vi "Build Toolkit HTML Documentation.vi"(8 "Error In":errorcluster) -> (0 "Error Out":errorcluster)   [LabVIEW 2018, in "Scripts.lvlib"]
uses:
  Scripts.lvlib
  <vilib>/Field R&D Services/Labricator/Toolkit/Labricator.lvlib
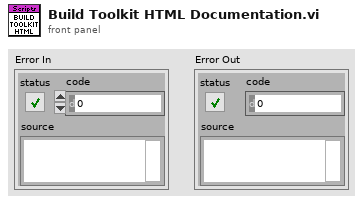
[diagram p1: front panel]
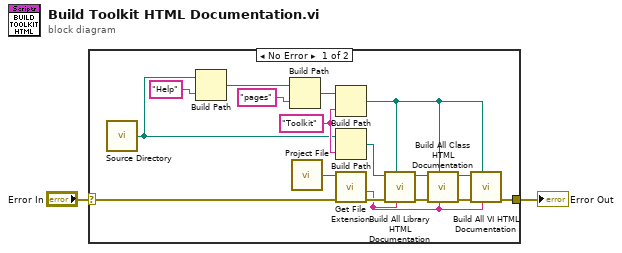
[diagram p0: block diagram]
diagram:
  n1 = case shown="No Error" "Error In" {
    selector: "Error In" -> [w14 w20]
    tunnel: [w17 w20] -> w1
    frame No Error {
      w7 = "Toolkit" ("name or relative path")
      n2 = call <vilib>:"Source Directory.vi"() -> ("Source Directory"=w5:path)
      n3 = Build Path(base path=w5, name or relative path="Help") -> (appended path=w10:path)
      n4 = Build Path(base path=w10, name or relative path="pages") -> (appended path=w8:path)
      n5 = call <vilib>:"Project File.vi"() -> ("Project File"=w15:path)
      n6 = Build Path(base path=w8, name or relative path=w7) -> (appended path=w6:path)
      n7 = Build Path(base path=w5, name or relative path=w7) -> (appended path=w16:path)
      n8 = call <vilib>:"Get File Extension.vi"("error in (no error)"=w14, "file"=w15) -> ("error out"=w13:errorcluster, "filename without extension"=w12:string)  [unwired: 5 in, 3 out]
      n9 = call "Build All Library HTML Documentation.vi"("Requirement"=w12, "Destination"=w6, "Error In"=w13, "Source In"=w16) -> ("Error Out"=w18:errorcluster, "Source Out"=w19:path)  [unwired: 6 in]
      n10 = call "Build All Class HTML Documentation.vi"("Requirement"=w12, "Destination"=w6, "Error In"=w18, "Source In"=w19) -> ("Error Out"=w3:errorcluster, "Source Out"=w4:path)  [unwired: 6 in]
      n11 = call "Build All VI HTML Documentation.vi"("Requirement"=w12, "Destination"=w6, "Error In"=w3, "Source In"=w4) -> ("Error Out"=w17:errorcluster)  [unwired: 6 in, 1 out]
    }
    frame Error {
    }
  }
  "Error Out" <- w1
